vi "Read from Driver.vi"(8 "error in":errorcluster, 11 "Signal Indices Out":i32[](array[numeric])) -> (0 "error out":errorcluster, 3 "Driver Values":i32[](array[numeric]))   [LabVIEW 2026, in "Runtime Configuration Support Inline Async Example Custom Device Engine.lvlib"]
uses:
  Runtime Configuration Support Inline Async Example Custom Device Engine.lvlib
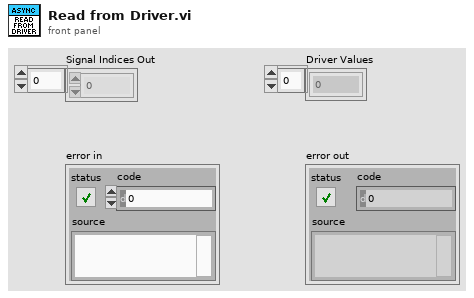
[diagram p1: front panel]
types:
  T1 = enum16{"Initialize", "Set In Val", "Get In Val", "Set Block", "Set Out Val", "Get Out Val", "Get In Array", "Get Out Array"}
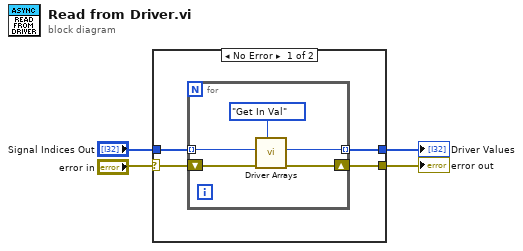
[diagram p0: block diagram]
diagram:
  n1 = case shown="No Error" "error in" {
    selector: "error in" -> [w7 w14]
    tunnel: "Signal Indices Out" -> [w6 _]
    tunnel: [w5 _] -> w1
    tunnel: [w8 w14] -> w4
    frame No Error {
      n2 = for {
        tunnel: w6 -> [w11] mode=indexing
        tunnel: [w9] -> w5 mode=indexing
        shift-right: [w12] -> w8
        shift-left: w7 -> [w13]
        n3 = call "Driver Arrays.vi"("error in"=w13, "Index"=w11, "Curr Operation"=T1."Get In Val") -> ("error out"=w12:errorcluster, "Value"=w9:i32)  [unwired: 5 in, 2 out]
      }
    }
    frame Error {
    }
  }
  "Driver Values" <- w1
  "error out" <- w4
